vi "ImageFrameCatchUp.vi"(6 "Frame Diff Limit":i32, 7 "Images Acquired":i32, 8 "error in (no error)":errorcluster, 9 "Enable":bool, 11 "Image in":refnum<class "Image.lvclass">) -> (0 "error out":errorcluster, 1 "Frames Skipped":i32, 3 "Image out":refnum<class "Image.lvclass">)   [LabVIEW 2012, in "Image.lvclass"]
uses:
  classes/Image.lvclass
  typedefs/ScanMode.ctl
  classes/Image.lvclass/Image.ctl
panel:
  out "size(s)":i32[](array[numeric])
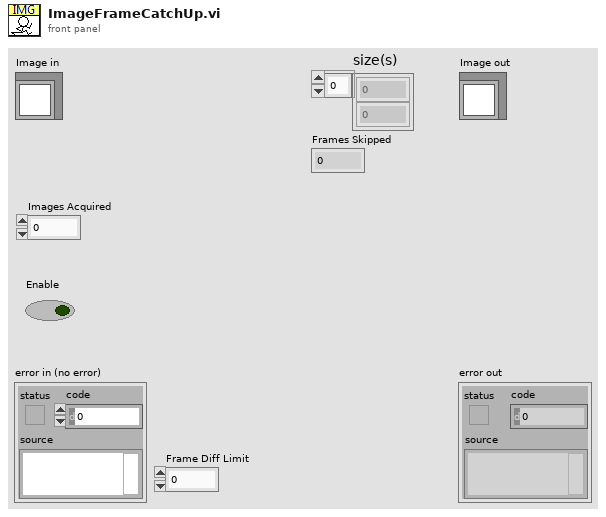
[diagram p1: front panel]
types:
  T1 = typedef "ScanMode.ctl" = enum16{"None", "Continuous", "Point Scan (CH3 cursor)", "Point Scan Move (CH3 cursor)", "Grab", "Grab Move Stage", "Grab Move Z-stage", "Cont. Move Z-stage", "Spec Move Stage", "Spec Move Cont", "Surf Calib"}
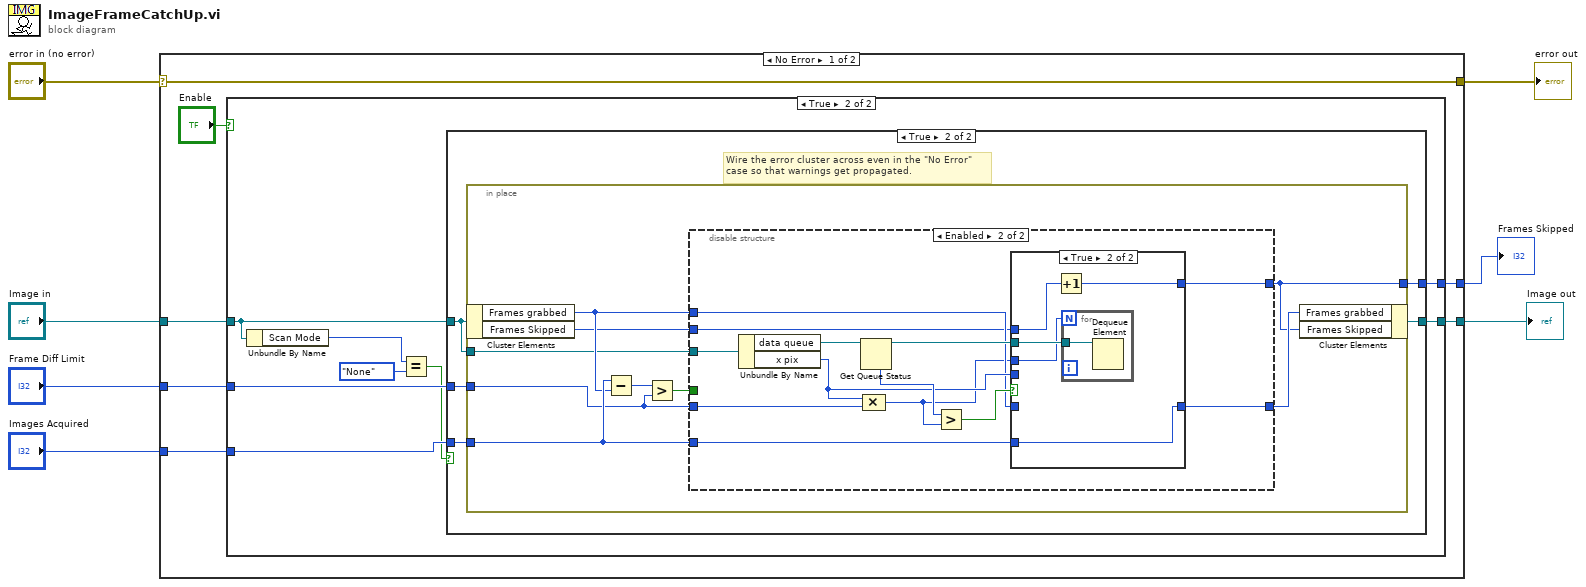
[diagram p0: block diagram]
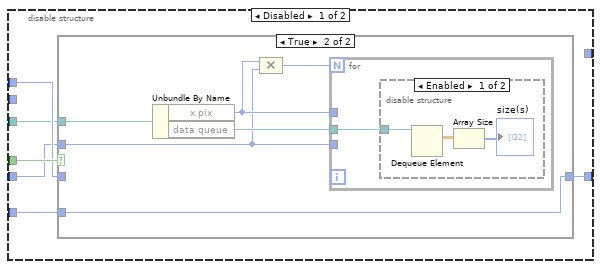
[diagram p4: hidden frame]
diagram:
  n1 = case shown="No Error" "error in (no error)" {
    selector: "error in (no error)" -> [w14 w78]
    tunnel: [w14 w78] -> w6
    tunnel: [w11 w77] -> w4
    tunnel: "Image in" -> [w10 w77]
    tunnel: "Images Acquired" -> [w13 _]
    tunnel: "Frame Diff Limit" -> [w12 _]
    tunnel: [w8 _] -> w1
    frame No Error {
      n2 = case shown="True" "Enable" {
        tunnel: w13 -> [_ w23]
        tunnel: w12 -> [_ w22]
        tunnel: [w15 w21] -> w11
        tunnel: w10 -> [w15 w20]
        tunnel: [_ w16] -> w8
        frame False {
        }
        frame True {
          n3 = Unbundle By Name(w20) -> ("Scan Mode"=w19:T1)
          n4 = Equal?(x=w19, y=ScanMode."None") -> (x = y?=w17:bool)
          n5 = case shown="True" w17 {
            tunnel: w23 -> [_ w29]
            tunnel: w22 -> [_ w28]
            tunnel: [w24 w27] -> w21
            tunnel: w20 -> [w24 w26]
            tunnel: [_ w25] -> w16
            frame False {
            }
            frame True {
              # "Wire the error cluster across even in the \"No Error\"\ncase so that warnings get propagated."
              n6 = in-place {
                in-place-border: w29 -> [w37]
                in-place-border: w28 -> [w32]
                in-place-border: w26 -> [w33]
                in-place-border: [w30] -> w25
                n7 = in-place-cluster #1(w26) -> ("Frames grabbed"=w35:i32, "Frames Skipped"=w31:i32)
                n8 = Subtract(x=w37, y=w35) -> (x-y=w34:i32)
                n9 = Greater?(x=w34, y=w32) -> (0:w38:bool)
                n10 = disable-structure shown="Enabled" {
                  disable-tunnel: w38 -> [w44 _]
                  disable-tunnel: w37 -> [w43 w60]
                  disable-tunnel: [w42 w61] -> w36
                  disable-tunnel: w35 -> [w41 w59]
                  disable-tunnel: w33 -> [w40 w68]
                  disable-tunnel: w32 -> [w39 w66]
                  disable-tunnel: w31 -> [_ w58]
                  disable-tunnel: [_ w57] -> w30
                  frame Disabled {
                    n11 = case shown="True" w44 {
                      tunnel: w43 -> [_ w48]
                      tunnel: [w45 w48] -> w42
                      tunnel: w41 -> [w45 _]
                      tunnel: w40 -> [_ w51]
                      tunnel: w39 -> [_ w46]
                      frame False {
                      }
                      frame True {
                        n12 = Unbundle By Name(w51) -> ("x pix"=w47:i32, "data queue"=w50:refnum<queue>)
                        n13 = Compound Arithmetic op=MULTIPLY(w47, w46) -> (w49:i32)
                        n14 = for {
                          N: w49 -> [_]
                          tunnel: w50 -> [w52]
                          tunnel: w46 -> [_]
                          tunnel: w47 -> [_]
                          n15 = disable-structure shown="Enabled" {
                            disable-tunnel: w52 -> [w55 _]
                            frame Enabled {
                              n16 = Dequeue Element(queue=w55) -> (element=w54:dbl[][])  [unwired: 2 in, 3 out]
                              n17 = Array Size(array=w54) -> (size(s)=→"size(s)":i32[])
                            }
                            frame Disabled {
                            }
                          }
                        }
                      }
                    }
                  }
                  frame Enabled {
                    n18 = Unbundle By Name(w68) -> ("data queue"=w67:refnum<queue>, "x pix"=w62:i32)
                    n19 = Get Queue Status(queue=w67) -> (queue out=w63:refnum<queue>, # elements in queue=w65:i32)  [unwired: 2 in, 6 out]
                    n20 = Compound Arithmetic op=MULTIPLY(w62, w66) -> (w56:i32)
                    n21 = Greater?(x=w65, y=w56) -> (0:w64:bool)
                    n22 = case shown="True" w64 {
                      tunnel: w63 -> [_ w75]
                      tunnel: w62 -> [_ _]
                      tunnel: [w70 w74] -> w61
                      tunnel: w60 -> [_ w74]
                      tunnel: w59 -> [w70 _]
                      tunnel: w58 -> [w69 w73]
                      tunnel: [w69 w72] -> w57
                      tunnel: w56 -> [_ w71]
                      frame False {
                      }
                      frame True {
                        n23 = Increment(x=w73) -> (x+1=w72:i32)
                        n24 = for {
                          N: w71 -> [_]
                          tunnel: w75 -> [w76]
                          n25 = Dequeue Element(queue=w76) -> ()  [unwired: 2 in, 4 out]
                        }
                      }
                    }
                  }
                }
                n26 = in-place-cluster #1("Frames grabbed"=w36, "Frames Skipped"=w30) -> (w27:refnum<class "Image.lvclass">)
              }
            }
          }
        }
      }
    }
    frame Error {
    }
  }
  "error out" <- w6
  "Image out" <- w4
  "Frames Skipped" <- w1
